vi "Stop.vi"(8 "error in":errorcluster, 11 "CFG Base in":refnum<class "CFG Base.lvclass">) -> (0 "error out":errorcluster, 3 "CFG Base out":refnum<class "CFG Base.lvclass">)   [LabVIEW 2023, in "HAL.lvlib" / "CFG Base.lvclass"]
uses:
  CFG Base.lvclass
  CFG Base.lvclass/CFG Base.ctl
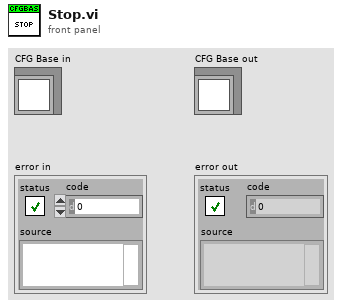
[diagram p1: front panel]
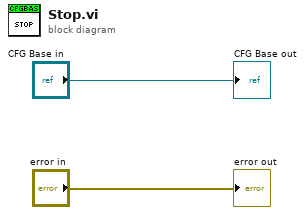
[diagram p0: block diagram]
diagram:
  "error out" <- "error in"
  "CFG Base out" <- "CFG Base in"
